vi "Build analog value array.vi"(0 "System no.":i32=1 min=1 step=1, 1 "Absolute (T)/Relative":bool=TRUE, 2 "String":string, 3 "Initialize":bool, 4 "Values in":dbl[](array[numeric]) format="%.8f", 5 "error in":errorcluster, 6 "Waveform?":bool, 7 "Voltage?":bool=TRUE, 8 "W_Wave?":bool, 9 "Waveform to write":waveform(dbl)[](array[waveform]), 10 "Range check?":bool=TRUE) -> (14 "Values out":dbl[](array[numeric]) format="%.8f", 15 "Axes out":string[](array[string]), 16 "Waveform out":waveform(dbl)[](array[waveform]), 17 "T":dbl[](array[numeric]), 19 "error out":errorcluster)   [LabVIEW 2020]
doc: "This vi returns an array of numbers or waveforms and axes parsed from \"String\", which must follow the GCS 2.0 conventions. If Initialize? is TRUE, the VI is initialized with Values in. If Absolute (T)/Relative is TRUE, the values in String are considered to be absolute position values, for FALSE they are considered relative to the current voltage/position. If Voltage? is FALSE, the conversion factor V/µm is read from GlobalAnalog.vi, the values in String are considered to be position values and Values o ut/Waveform out contains voltage information. If Voltage? is TRUE, the values in String are considered to be voltage values. T is the total time for Waveform out. \n\nValid for Analog systems."
uses:
  Global Analog.vi
  NI_MAPro.lvlib
panel:
  # "This vi returns an array of numbers or waveforms and axes parsed from \"String\" which must follow the GCS 2.0 conventions. If Initialize? is TRUE, the VI is initialized with Values in. If\nAbsolute (T)/Relative is TRUE, the values in String are considered to be absolute position values, for FALSE relative position values. If Voltage? is FALSE, the conversion factor V/µm is \nread from GlobalAnalog.vi, the values in String are considered to be position values and Values out/Waveform out contains voltage information. T is the total time for Waveform out."
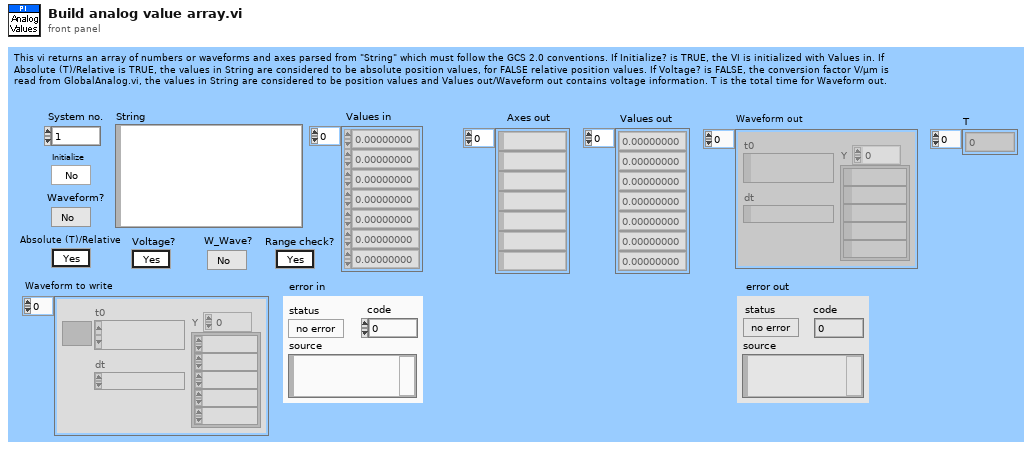
[diagram p1: front panel]
types:
  T1 = cluster{"Conversion factor":dbl[], "Velocity":dbl[], "Velocity control mode":bool, "AO.Resolution":dbl, "Lower voltage limit (V)":dbl, "Upper voltage limit (V)":dbl, "AO_WF_T (s)":dbl, "AI Sample Rate":dbl, "AI Samples/Channel":i32, "Hyperbit":bool, "Offset (V)":dbl[], "Hyperbit StayOnPos":bool, "Gain (V)":dbl[], "Bit rate (Hz)":dbl, "PWM rate (Hz)":dbl, "HyperBit Password":string, "AO.MaxRate":dbl, "Conversion offset":dbl[]}[]
  T2 = cluster{"Conversion factor":dbl[], "Velocity":dbl[], "Velocity control mode":bool, "AO.Resolution":dbl, "Lower voltage limit (V)":dbl, "Upper voltage limit (V)":dbl, "AO_WF_T (s)":dbl, "AI Sample Rate":dbl, "AI Samples/Channel":i32, "Hyperbit":bool, "Offset (V)":dbl[], "Hyperbit StayOnPos":bool, "Gain (V)":dbl[], "Bit rate (Hz)":dbl, "PWM rate (Hz)":dbl, "HyperBit Password":string, "AO.MaxRate":dbl, "Conversion offset":dbl[]}
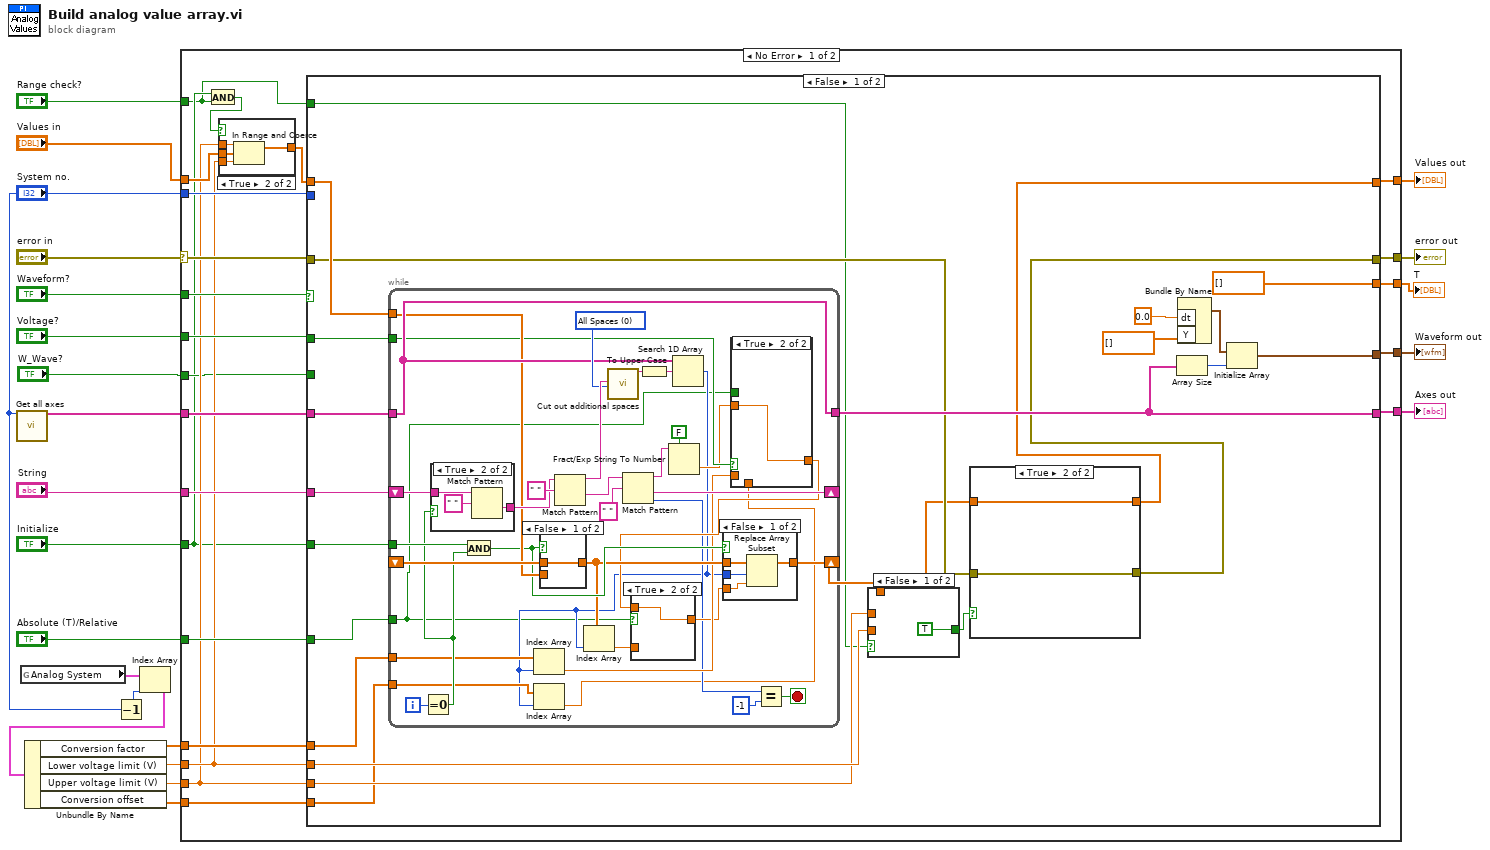
[diagram p0: block diagram]
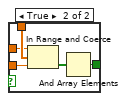
[diagram p3: hidden frame]
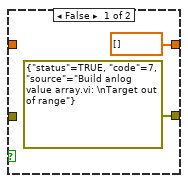
[diagram p4: hidden frame]
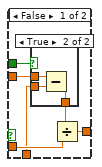
[diagram p5: hidden frame]
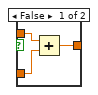
[diagram p7: hidden frame]
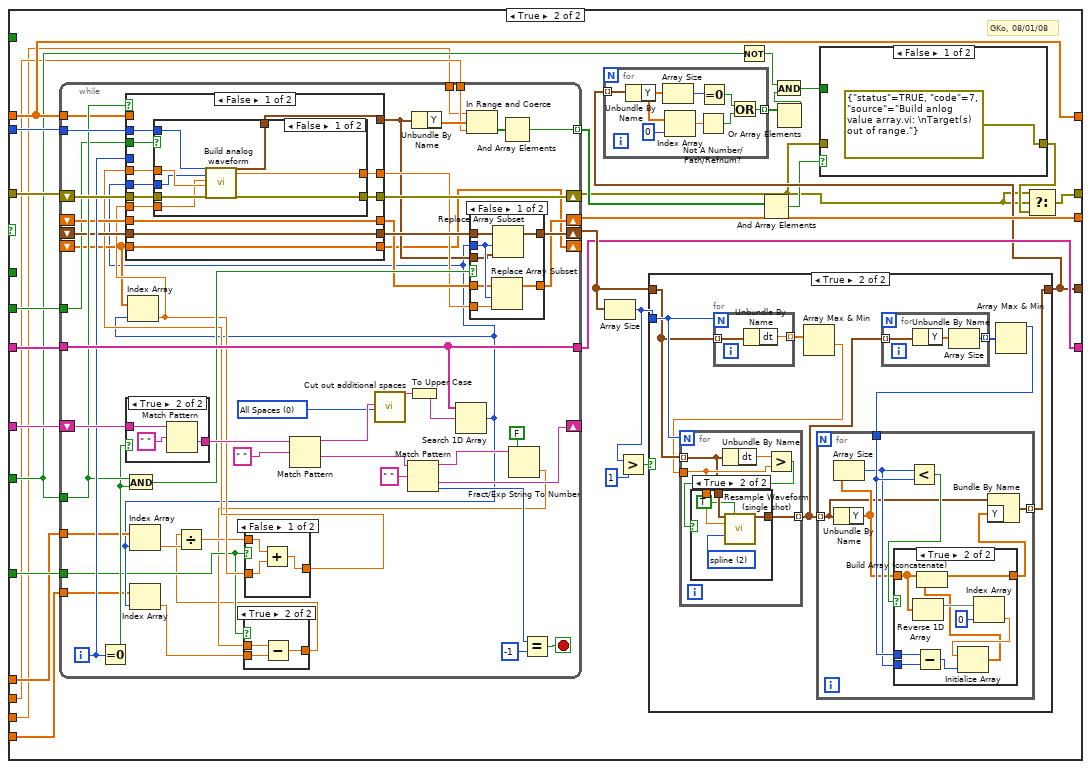
[diagram p11: hidden frame]
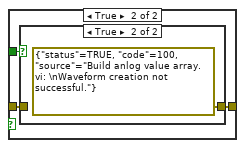
[diagram p12: hidden frame]
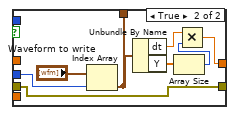
[diagram p20: hidden frame]
diagram:
  n1 = call "Get all axes.vi"("System no."="System no.") -> ("Conn. Axes"=w22:string[])  [unwired: 18 out]
  n2 = global read "Global Analog.vi" "Analog System"() -> (w8:T1)
  n3 = Decrement(x="System no.") -> (x-1=w9:i32)
  n4 = Index Array(array=w8, index=w9) -> (element=w10:T2)
  n5 = Unbundle By Name(w10) -> ("Conversion factor"=w6:dbl[], "Lower voltage limit (V)"=w5:dbl, "Upper voltage limit (V)"=w4:dbl, "Conversion offset"=w1:dbl[])
  n6 = case shown="No Error" "error in" {
    selector: "error in" -> [w39 w352]
    tunnel: "String" -> [w45 _]
    tunnel: w22 -> [w44 w349]
    tunnel: [w43 string[] [] ("Conn. Axes")] -> w21
    tunnel: "Initialize" -> [w27 _]
    tunnel: [w42 dbl[] [] ("Values in")] -> w19
    tunnel: "Waveform?" -> [w41 _]
    tunnel: [w38 w352] -> w16
    tunnel: "System no." -> [w40 _]
    tunnel: "Values in" -> [w33 _]
    tunnel: "Absolute (T)/Relative" -> [w37 _]
    tunnel: [w36 w346] -> w13
    tunnel: [w35 dbl[] []] -> w12
    tunnel: "Voltage?" -> [w34 _]
    tunnel: w6 -> [w32 _]
    tunnel: w5 -> [w31 _]
    tunnel: w4 -> [w30 _]
    tunnel: "W_Wave?" -> [w28 _]
    tunnel: "Range check?" -> [w25 _]
    tunnel: w1 -> [w24 _]
    frame No Error {
      n7 = And(x=w27, y=w25) -> (x .and. y?=w26:bool)
      n8 = case shown="True" w26 {
        tunnel: w33 -> [w46 w50]
        tunnel: w31 -> [_ w49]
        tunnel: w30 -> [_ w48]
        tunnel: [w46 w47] -> w29
        frame False {
        }
        frame True {
          n9 = In Range and Coerce(upper limit=w48, x=w50, lower limit=w49) -> (coerced(x)=w47:dbl[])  [unwired: 1 out]
        }
      }
      n10 = case shown="False" w41 {
        tunnel: w45 -> [w73 w172]
        tunnel: [w56 w169] -> w42
        tunnel: w44 -> [w72 w171]
        tunnel: [w65 w162] -> w43
        tunnel: w27 -> [w71 w156]
        tunnel: w40 -> [_ w164]
        tunnel: w39 -> [w59 w170]
        tunnel: [w58 w146] -> w38
        tunnel: w29 -> [w70 w169]
        tunnel: w37 -> [w63 w163]
        tunnel: [w64 w158] -> w36
        tunnel: [dbl[] [] w161] -> w35
        tunnel: w34 -> [w61 _]
        tunnel: w32 -> [w55 w160]
        tunnel: w31 -> [w54 w152]
        tunnel: w30 -> [w53 w151]
        tunnel: w28 -> [_ w159]
        tunnel: w25 -> [w52 _]
        tunnel: w24 -> [w51 w145]
        frame False {
          n11 = while {
            shift-right: [w109] -> _
            shift-left: w73 -> [w118]
            shift-right: [w104] -> w57
            shift-left: _ -> [w102]
            tunnel: w72 -> [w103]
            tunnel: [w103] -> w65
            tunnel: w71 -> [w100]
            tunnel: w70 -> [w101]
            tunnel: w63 -> [w84]
            tunnel: w61 -> [w94]
            tunnel: w55 -> [w95]
            tunnel: w51 -> [w87]
            i -> [w107]
            stop <- w108 stop-if-true
            w112 = u16 0 items=["All Spaces", "Only if 1st char.", "Only if last char.", "Only if near \"=\"", "Only if 1st or last char.", "Only multiple"] ("Mode")
            n12 = Equal To 0?(x=w107) -> (x = 0?=w99:bool)
            n13 = case shown="True" w99 {
              tunnel: w118 -> [w141 w144]
              tunnel: [w141 w142] -> w116
              frame False {
              }
              frame True {
                n14 = Match Pattern(string=w144, regular expression=" ") -> (after substring=w142:string)  [unwired: 4 out]
              }
            }
            n15 = And(x=w100, y=w99) -> (x .and. y?=w98:bool)
            n16 = case shown="False" w98 {
              tunnel: [w139 w140] -> w96
              tunnel: w102 -> [w139 _]
              tunnel: w101 -> [_ w140]
              frame False {
              }
              frame True {
              }
            }
            n17 = Match Pattern(string=w116, regular expression=" ") -> (before substring=w113:string, after substring=w114:string)  [unwired: 3 out]
            n18 = call "Cut out additional spaces.vi"("String"=w113, "Mode"=w112) -> ("String out"=w106:string)  [unwired: 17 out]
            n19 = Match Pattern(string=w114, regular expression=" ") -> (before substring=w110:string, after substring=w109:string, offset past match=w90:i32)  [unwired: 2 out]
            n20 = To Upper Case(1:w106) -> (0:w88:string)
            n21 = Fract/Exp String To Number(use system decimal point (T)=FALSE, string=w110) -> (number=w89:dbl)  [unwired: 3 out]
            n22 = Search 1D Array(1D array=w103, element=w88) -> (index of element=w86:i32)  [unwired: 1 out]
            n23 = Index Array(array=w95, index=w86) -> (element=w92:dbl)
            n24 = Index Array(array=w87, index=w86) -> (element=w85:dbl)
            n25 = Index Array(array=w96, index=w86) -> (element=w97:dbl)
            n26 = case shown="True" w94 {
              tunnel: w89 -> [w122 w129]
              tunnel: [w124 w129] -> w93
              tunnel: w92 -> [w123 _]
              tunnel: w85 -> [w120 _]
              tunnel: w84 -> [w119 _]
              frame False {
                n27 = case shown="True" w119 {
                  tunnel: w122 -> [w125 w128]
                  tunnel: [w125 w127] -> w121
                  tunnel: w120 -> [_ w126]
                  frame False {
                  }
                  frame True {
                    n28 = Subtract(x=w128, y=w126) -> (x-y=w127:dbl)
                  }
                }
                n29 = Divide(x=w121, y=w123) -> (x/y=w124:dbl)
              }
              frame True {
              }
            }
            n30 = case shown="True" w84 {
              tunnel: w93 -> [w132 w133]
              tunnel: [w130 w133] -> w91
              tunnel: w97 -> [w131 _]
              frame False {
                n31 = Add(x=w132, y=w131) -> (x+y=w130:dbl)
              }
              frame True {
              }
            }
            n32 = case shown="False" w98 {
              tunnel: w86 -> [w137 _]
              tunnel: w91 -> [w136 _]
              tunnel: [w135 w138] -> w104
              tunnel: w96 -> [w134 w138]
              frame False {
                n33 = Replace Array Subset(array=w134, new element=w136, index=w137) -> (w135:dbl[])
              }
              frame True {
              }
            }
            n34 = Equal?(x=w90, y=-1) -> (x = y?=w108:bool)
          }
          n35 = case shown="False" w52 {
            tunnel: [TRUE w78] -> w60
            tunnel: w57 -> [_ w77]
            tunnel: w54 -> [_ w76]
            tunnel: w53 -> [_ w75]
            frame False {
            }
            frame True {
              n36 = In Range and Coerce(upper limit=w75, x=w77, lower limit=w76) -> (In Range?=w79:bool[])  [unwired: 1 out]
              n37 = And Array Elements(Boolean array=w79) -> (logical AND=w78:bool)
            }
          }
          n38 = case shown="True" w60 {
            tunnel: w59 -> [_ w83]
            tunnel: [errorcluster {"status"=TRUE, "code"=7, "source"="Build anlog value array.vi: \nTarget out of range"} ("error out") w83] -> w58
            tunnel: w57 -> [_ w82]
            tunnel: [dbl[] [] ("Values in") w82] -> w56
            frame False {
            }
            frame True {
            }
          }
          n39 = Array Size(array=w65) -> (size(s)=w66:i32)
          n40 = Bundle By Name("dt"=0.0, "Y"=dbl[] []) -> (w67:waveform(dbl))  [unwired: 1 out]
          n41 = Initialize Array(w67, w66) -> (w64:waveform(dbl)[])
        }
        frame True {
          # "GKo, 08/01/08"
          n42 = while {
            shift-right: [w270] -> _
            shift-left: w172 -> [w279]
            shift-right: [w265] -> w168
            shift-left: _ -> [w252]
            tunnel: w171 -> [w264]
            tunnel: [w264] -> w162
            tunnel: w156 -> [w258]
            tunnel: w164 -> [w261]
            tunnel: w169 -> [w255]
            shift-right: [w253] -> w161
            shift-left: _ -> [w251]
            tunnel: w160 -> [w249]
            shift-right: [w236] -> _
            shift-left: _ -> [w237]
            shift-right: [w262] -> w147
            shift-left: w170 -> [w263]
            tunnel: w163 -> [w232]
            tunnel: w159 -> [w244]
            tunnel: w152 -> [w240]
            tunnel: w151 -> [w239]
            tunnel: [w238] -> w150 mode=indexing
            tunnel: w145 -> [w234]
            i -> [w259]
            stop <- w268 stop-if-true
            w273 = u16 0 items=["All Spaces", "Only if 1st char.", "Only if last char.", "Only if near \"=\"", "Only if 1st or last char.", "Only multiple"] ("Mode")
            n43 = Equal To 0?(x=w259) -> (x = 0?=w257:bool)
            n44 = case shown="True" w257 {
              tunnel: w279 -> [w341 w344]
              tunnel: [w341 w342] -> w277
              frame False {
              }
              frame True {
                n45 = Match Pattern(string=w344, regular expression=" ") -> (after substring=w342:string)  [unwired: 4 out]
              }
            }
            n46 = And(x=w258, y=w257) -> (x .and. y?=w256:bool)
            n47 = Match Pattern(string=w277, regular expression=" ") -> (before substring=w274:string, after substring=w275:string)  [unwired: 3 out]
            n48 = call "Cut out additional spaces.vi"("String"=w274, "Mode"=w273) -> ("String out"=w267:string)  [unwired: 17 out]
            n49 = Match Pattern(string=w275, regular expression=" ") -> (before substring=w271:string, after substring=w270:string, offset past match=w269:i32)  [unwired: 2 out]
            n50 = To Upper Case(1:w267) -> (0:w245:string)
            n51 = Search 1D Array(1D array=w264, element=w245) -> (index of element=w235:i32)  [unwired: 1 out]
            n52 = Index Array(array=w237, index=w235) -> (element=w246:dbl)
            n53 = Index Array(array=w249, index=w235) -> (element=w248:dbl)
            n54 = Index Array(array=w234, index=w235) -> (element=w230:dbl)
            n55 = Fract/Exp String To Number(use system decimal point (T)=FALSE, string=w271) -> (number=w231:dbl)  [unwired: 3 out]
            n56 = case shown="True" w232 {
              tunnel: w231 -> [w280 w283]
              tunnel: w230 -> [_ w282]
              tunnel: [w280 w281] -> w229
              frame False {
              }
              frame True {
                n57 = Subtract(x=w283, y=w282) -> (x-y=w281:dbl)
              }
            }
            n58 = Divide(x=w229, y=w248) -> (x/y=w233:dbl)
            n59 = case shown="False" w232 {
              tunnel: w233 -> [w286 w287]
              tunnel: [w284 w287] -> w247
              tunnel: w246 -> [w285 _]
              frame False {
                n60 = Add(x=w286, y=w285) -> (x+y=w284:dbl)
              }
              frame True {
              }
            }
            n61 = case shown="False" w258 {
              tunnel: w263 -> [w308 w333]
              tunnel: w247 -> [w307 _]
              tunnel: [w306 w332] -> w262
              tunnel: [w301 w329] -> w254
              tunnel: w261 -> [w305 w331]
              tunnel: w235 -> [w304 _]
              tunnel: w246 -> [w303 _]
              tunnel: [w302 w328] -> w260
              tunnel: w259 -> [_ _]
              tunnel: w255 -> [_ w325]
              tunnel: w252 -> [w302 _]
              tunnel: w251 -> [w301 _]
              tunnel: [w300 w327] -> w243
              tunnel: [w299 w326] -> w250
              tunnel: [w298 w325] -> w236
              tunnel: w237 -> [w298 _]
              tunnel: w244 -> [w297 _]
              frame False {
                n62 = case shown="False" w297 {
                  tunnel: w308 -> [w316 w322]
                  tunnel: w307 -> [w315 _]
                  tunnel: [w314 w322] -> w306
                  tunnel: w305 -> [w313 _]
                  tunnel: w304 -> [w312 w324]
                  tunnel: w303 -> [w311 _]
                  tunnel: [w310 w321] -> w300
                  tunnel: [w309 w317] -> w299
                  frame False {
                    n63 = call "Build analog waveform.vi"("System no."=w313, "Index of axis"=w312, "Start voltage"=w311, "Target voltage"=w315, "error in"=w316) -> ("Waveform"=w310:waveform(dbl), "T (s)"=w309:dbl, "error out"=w314:errorcluster)  [unwired: 12 out]
                  }
                  frame True {
                    n64 = Index Array(array="Waveform to write", index=w324) -> (element=w321:waveform(dbl))
                    n65 = Unbundle By Name(w321) -> ("dt"=w319:dbl, "Y"=w320:dbl[])
                    n66 = Array Size(array=w320) -> (size(s)=w318:i32)
                    n67 = Multiply(x=w319, y=w318) -> (x*y=w317:dbl)
                  }
                }
              }
              frame True {
                n68 = Array Size(array=w325) -> (size(s)=w330:i32)
                n69 = for {
                  N: w330 -> [_]
                  tunnel: [w334] -> w329 mode=indexing
                  tunnel: w331 -> [w338]
                  tunnel: [w335] -> w328 mode=indexing
                  shift-right: [w339] -> w332
                  shift-left: w333 -> [w340]
                  tunnel: w325 -> [w337] mode=indexing
                  tunnel: [w335] -> w327
                  tunnel: [w334] -> w326
                  i -> [w336]
                  n70 = call "Build analog waveform.vi"("System no."=w338, "Index of axis"=w336, "Start voltage"=w337, "Target voltage"=w337, "error in"=w340) -> ("Waveform"=w335:waveform(dbl), "T (s)"=w334:dbl, "error out"=w339:errorcluster)  [unwired: 12 out]
                }
              }
            }
            n71 = Unbundle By Name(w243) -> ("Y"=w241:dbl[])
            n72 = In Range and Coerce(upper limit=w239, x=w241, lower limit=w240) -> (In Range?=w242:bool[])  [unwired: 1 out]
            n73 = case shown="False" w256 {
              tunnel: [w294 w295] -> w265
              tunnel: [w293 w296] -> w253
              tunnel: w254 -> [w289 w296]
              tunnel: w235 -> [w292 _]
              tunnel: w260 -> [w291 w295]
              tunnel: w243 -> [w290 _]
              tunnel: w250 -> [w288 _]
              frame False {
                n74 = Replace Array Subset(array=w289, new element=w288, index=w292) -> (w293:dbl[])
                n75 = Replace Array Subset(array=w291, new element=w290, index=w292) -> (w294:waveform(dbl)[])
              }
              frame True {
              }
            }
            n76 = And Array Elements(Boolean array=w242) -> (logical AND=w238:bool)
            n77 = Equal?(x=w269, y=-1) -> (x = y?=w268:bool)
          }
          n78 = Array Size(array=w168) -> (size(s)=w166:i32)
          n79 = Greater?(x=w166, y=1) -> (0:w167:bool)
          n80 = case shown="True" w167 {
            tunnel: w166 -> [_ w195]
            tunnel: w168 -> [w187 w194]
            tunnel: [w187 w191] -> w158
            frame False {
            }
            frame True {
              n81 = for {
                N: w195 -> [_]
                tunnel: w194 -> [w228] mode=indexing
                tunnel: [w227] -> w193 mode=indexing
                n82 = Unbundle By Name(w228) -> ("dt"=w227:dbl)
              }
              n83 = Array Max & Min(array=w193) -> (min value=w192:dbl)  [unwired: 3 out]
              n84 = for {
                N: w195 -> [_]
                tunnel: w194 -> [w217] mode=indexing
                tunnel: [w216] -> w188 mode=indexing
                tunnel: w192 -> [w218]
                n85 = Unbundle By Name(w217) -> ("dt"=w220:dbl)
                n86 = Greater?(x=w220, y=w218) -> (0:w219:bool)
                n87 = case shown="True" w219 {
                  tunnel: [w221 w223] -> w216
                  tunnel: w217 -> [w221 w225]
                  tunnel: w218 -> [_ w224]
                  frame False {
                  }
                  frame True {
                    w226 = u16 2 items=["coerce", "linear", "spline", "FIR filter"] ("interpolation mode")
                    n88 = call "Resample Waveform (single shot).vi"("waveform in"=w225, "open interval? (F)"=TRUE, "dt"=w224, "interpolation mode"=w226) -> ("resampled waveform out"=w223:waveform(dbl))  [unwired: 8 in, 3 out]
                  }
                }
              }
              n89 = for {
                tunnel: w188 -> [w198] mode=indexing
                tunnel: [w196] -> w189 mode=indexing
                n90 = Unbundle By Name(w198) -> ("Y"=w197:dbl[])
                n91 = Array Size(array=w197) -> (size(s)=w196:i32)
              }
              n92 = Array Max & Min(array=w189) -> (max value=w190:i32)  [unwired: 3 out]
              n93 = for {
                tunnel: w190 -> [w204]
                tunnel: [w201] -> w191 mode=indexing
                tunnel: w188 -> [w199] mode=indexing
                n94 = Unbundle By Name(w199) -> ("Y"=w200:dbl[])
                n95 = Array Size(array=w200) -> (size(s)=w203:i32)
                n96 = Less?(x=w203, y=w204) -> (x < y?=w205:bool)
                n97 = case shown="True" w205 {
                  tunnel: w200 -> [w206 w215]
                  tunnel: w204 -> [_ w211]
                  tunnel: w203 -> [_ w210]
                  tunnel: [w206 w207] -> w202
                  frame False {
                  }
                  frame True {
                    n98 = Reverse 1D Array(array=w215) -> (reversed array=w214:dbl[])
                    n99 = Subtract(x=w211, y=w210) -> (x-y=w209:i32)
                    n100 = Index Array(array=w214, index=0) -> (element=w212:dbl)
                    n101 = Initialize Array(w212, w209) -> (w208:dbl[])
                    n102 = Build Array (concatenate)(w215, w208) -> (w207:dbl[])
                  }
                }
                n103 = Bundle By Name(cluster=w199, "Y"=w202) -> (w201:waveform(dbl))
              }
            }
          }
          n104 = for {
            tunnel: w158 -> [w186] mode=indexing
            tunnel: [w179] -> w157 mode=indexing
            n105 = Unbundle By Name(w186) -> ("Y"=w183:dbl[])
            n106 = Array Size(array=w183) -> (size(s)=w185:i32)
            n107 = Index Array(array=w183, index=0) -> (element=w181:dbl)
            n108 = Not A Number/Path/Refnum?(number/path/refnum=w181) -> (NaN/Path/Refnum?=w180:bool)
            n109 = Equal To 0?(x=w185) -> (x = 0?=w184:bool)
            n110 = Or(x=w184, y=w180) -> (x .or. y?=w179:bool)
          }
          n111 = Not(x=w156) -> (.not. x?=w154:bool)
          n112 = And Array Elements(Boolean array=w150) -> (logical AND=w149:bool)
          n113 = Or Array Elements(Boolean array=w157) -> (logical OR=w155:bool)
          n114 = And(x=w154, y=w155) -> (x .and. y?=w153:bool)
          n115 = case shown="False" w149 {
            tunnel: w147 -> [_ w176]
            tunnel: [errorcluster {"status"=TRUE, "code"=7, "source"="Build anlog value array.vi: \nTarget(s) out of range."} ("error out") w175] -> w148
            tunnel: w153 -> [_ w174]
            frame False {
            }
            frame True {
              n116 = case shown="True" w174 {
                tunnel: w176 -> [w177 _]
                tunnel: [w177 errorcluster {"status"=TRUE, "code"=100, "source"="Build anlog value array.vi: \nWaveform creation not successful."} ("error out")] -> w175
                frame False {
                }
                frame True {
                }
              }
            }
          }
          n117 = Select(t=w147, s=w147, f=w148) -> (s? t:f=w146:errorcluster)
        }
      }
    }
    frame Error {
      n118 = Array Size(array=w349) -> (size(s)=w347:i32)
      n119 = Bundle By Name("dt"=0.0, "Y"=dbl[] []) -> (w348:waveform(dbl))  [unwired: 1 out]
      n120 = Initialize Array(w348, w347) -> (w346:waveform(dbl)[])
    }
  }
  "Values out" <- w19
  "Axes out" <- w21
  "error out" <- w16
  "Waveform out" <- w13
  "T" <- w12
